vi "SeqeunceDefinitionDialog.vi"(11 "TestSequence":T3[](array[typedef])) -> (1 "TestSequence out":T3[](array[typedef]), 3 "Cancelled?":bool=TRUE)   [LabVIEW 2017]
doc: "Use this template to create a dialog box with event handling."
uses:
  ModuleUICluster.ctl
  TestStep-StepType.ctl
  TestStepTypes.ctl
  RF Direction.ctl
  PolarizationSelect.ctl
panel:
  in  "Save As File":bool
  in  "Load File":bool
  in  "tab":T1(tab)
  in  "module 7":T2={"Tx Vertical"=FALSE, "Tx Horizontal"=FALSE, "Rx Vertical"=FALSE, "Rx Horizontal"=FALSE, "Attenuation, dB"=[63], "Phase Shift, deg"=[64]}
  in  "module 6":T2={"Tx Vertical"=FALSE, "Tx Horizontal"=FALSE, "Rx Vertical"=FALSE, "Rx Horizontal"=FALSE, "Attenuation, dB"=[63], "Phase Shift, deg"=[64]}
  in  "module 5":T2={"Tx Vertical"=FALSE, "Tx Horizontal"=FALSE, "Rx Vertical"=FALSE, "Rx Horizontal"=FALSE, "Attenuation, dB"=[63], "Phase Shift, deg"=[64]}
  in  "module 4":T2={"Tx Vertical"=FALSE, "Tx Horizontal"=FALSE, "Rx Vertical"=FALSE, "Rx Horizontal"=FALSE, "Attenuation, dB"=[63], "Phase Shift, deg"=[64]}
  in  "module 3":T2={"Tx Vertical"=FALSE, "Tx Horizontal"=FALSE, "Rx Vertical"=FALSE, "Rx Horizontal"=FALSE, "Attenuation, dB"=[63], "Phase Shift, deg"=[64]}
  in  "module 2":T2={"Tx Vertical"=FALSE, "Tx Horizontal"=FALSE, "Rx Vertical"=FALSE, "Rx Horizontal"=FALSE, "Attenuation, dB"=[63], "Phase Shift, deg"=[64]}
  in  "module 1":T2={"Tx Vertical"=FALSE, "Tx Horizontal"=FALSE, "Rx Vertical"=FALSE, "Rx Horizontal"=FALSE, "Attenuation, dB"=[63], "Phase Shift, deg"=[64]}
  in  "module 0":T2={"Tx Vertical"=FALSE, "Tx Horizontal"=FALSE, "Rx Vertical"=FALSE, "Rx Horizontal"=FALSE, "Attenuation, dB"=[63], "Phase Shift, deg"=[64]}
  in  "module 8":T2={"Tx Vertical"=FALSE, "Tx Horizontal"=FALSE, "Rx Vertical"=FALSE, "Rx Horizontal"=FALSE, "Attenuation, dB"=[63], "Phase Shift, deg"=[64]}
  in  "module 9":T2={"Tx Vertical"=FALSE, "Tx Horizontal"=FALSE, "Rx Vertical"=FALSE, "Rx Horizontal"=FALSE, "Attenuation, dB"=[63], "Phase Shift, deg"=[64]}
  in  "module 10":T2={"Tx Vertical"=FALSE, "Tx Horizontal"=FALSE, "Rx Vertical"=FALSE, "Rx Horizontal"=FALSE, "Attenuation, dB"=[63], "Phase Shift, deg"=[64]}
  in  "module 11":T2={"Tx Vertical"=FALSE, "Tx Horizontal"=FALSE, "Rx Vertical"=FALSE, "Rx Horizontal"=FALSE, "Attenuation, dB"=[63], "Phase Shift, deg"=[64]}
  in  "module 12":T2={"Tx Vertical"=FALSE, "Tx Horizontal"=FALSE, "Rx Vertical"=FALSE, "Rx Horizontal"=FALSE, "Attenuation, dB"=[63], "Phase Shift, deg"=[64]}
  in  "module 13":T2={"Tx Vertical"=FALSE, "Tx Horizontal"=FALSE, "Rx Vertical"=FALSE, "Rx Horizontal"=FALSE, "Attenuation, dB"=[63], "Phase Shift, deg"=[64]}
  in  "module 14":T2={"Tx Vertical"=FALSE, "Tx Horizontal"=FALSE, "Rx Vertical"=FALSE, "Rx Horizontal"=FALSE, "Attenuation, dB"=[63], "Phase Shift, deg"=[64]}
  in  "module 15":T2={"Tx Vertical"=FALSE, "Tx Horizontal"=FALSE, "Rx Vertical"=FALSE, "Rx Horizontal"=FALSE, "Attenuation, dB"=[63], "Phase Shift, deg"=[64]}
  in  "module 23":T2={"Tx Vertical"=FALSE, "Tx Horizontal"=FALSE, "Rx Vertical"=FALSE, "Rx Horizontal"=FALSE, "Attenuation, dB"=[63], "Phase Shift, deg"=[64]}
  in  "module 22":T2={"Tx Vertical"=FALSE, "Tx Horizontal"=FALSE, "Rx Vertical"=FALSE, "Rx Horizontal"=FALSE, "Attenuation, dB"=[63], "Phase Shift, deg"=[64]}
  in  "module 21":T2={"Tx Vertical"=FALSE, "Tx Horizontal"=FALSE, "Rx Vertical"=FALSE, "Rx Horizontal"=FALSE, "Attenuation, dB"=[63], "Phase Shift, deg"=[64]}
  in  "module 20":T2={"Tx Vertical"=FALSE, "Tx Horizontal"=FALSE, "Rx Vertical"=FALSE, "Rx Horizontal"=FALSE, "Attenuation, dB"=[63], "Phase Shift, deg"=[64]}
  in  "module 19":T2={"Tx Vertical"=FALSE, "Tx Horizontal"=FALSE, "Rx Vertical"=FALSE, "Rx Horizontal"=FALSE, "Attenuation, dB"=[63], "Phase Shift, deg"=[64]}
  in  "module 18":T2={"Tx Vertical"=FALSE, "Tx Horizontal"=FALSE, "Rx Vertical"=FALSE, "Rx Horizontal"=FALSE, "Attenuation, dB"=[63], "Phase Shift, deg"=[64]}
  in  "module 17":T2={"Tx Vertical"=FALSE, "Tx Horizontal"=FALSE, "Rx Vertical"=FALSE, "Rx Horizontal"=FALSE, "Attenuation, dB"=[63], "Phase Shift, deg"=[64]}
  in  "module 16":T2={"Tx Vertical"=FALSE, "Tx Horizontal"=FALSE, "Rx Vertical"=FALSE, "Rx Horizontal"=FALSE, "Attenuation, dB"=[63], "Phase Shift, deg"=[64]}
  in  "module 31":T2={"Tx Vertical"=FALSE, "Tx Horizontal"=FALSE, "Rx Vertical"=FALSE, "Rx Horizontal"=FALSE, "Attenuation, dB"=[63], "Phase Shift, deg"=[64]}
  in  "module 30":T2={"Tx Vertical"=FALSE, "Tx Horizontal"=FALSE, "Rx Vertical"=FALSE, "Rx Horizontal"=FALSE, "Attenuation, dB"=[63], "Phase Shift, deg"=[64]}
  in  "module 29":T2={"Tx Vertical"=FALSE, "Tx Horizontal"=FALSE, "Rx Vertical"=FALSE, "Rx Horizontal"=FALSE, "Attenuation, dB"=[63], "Phase Shift, deg"=[64]}
  in  "module 28":T2={"Tx Vertical"=FALSE, "Tx Horizontal"=FALSE, "Rx Vertical"=FALSE, "Rx Horizontal"=FALSE, "Attenuation, dB"=[63], "Phase Shift, deg"=[64]}
  in  "module 27":T2={"Tx Vertical"=FALSE, "Tx Horizontal"=FALSE, "Rx Vertical"=FALSE, "Rx Horizontal"=FALSE, "Attenuation, dB"=[63], "Phase Shift, deg"=[64]}
  in  "module 26":T2={"Tx Vertical"=FALSE, "Tx Horizontal"=FALSE, "Rx Vertical"=FALSE, "Rx Horizontal"=FALSE, "Attenuation, dB"=[63], "Phase Shift, deg"=[64]}
  in  "module 25":T2={"Tx Vertical"=FALSE, "Tx Horizontal"=FALSE, "Rx Vertical"=FALSE, "Rx Horizontal"=FALSE, "Attenuation, dB"=[63], "Phase Shift, deg"=[64]}
  in  "module 24":T2={"Tx Vertical"=FALSE, "Tx Horizontal"=FALSE, "Rx Vertical"=FALSE, "Rx Horizontal"=FALSE, "Attenuation, dB"=[63], "Phase Shift, deg"=[64]}
  in  "module 39":T2={"Tx Vertical"=FALSE, "Tx Horizontal"=FALSE, "Rx Vertical"=FALSE, "Rx Horizontal"=FALSE, "Attenuation, dB"=[63], "Phase Shift, deg"=[64]}
  in  "module 38":T2={"Tx Vertical"=FALSE, "Tx Horizontal"=FALSE, "Rx Vertical"=FALSE, "Rx Horizontal"=FALSE, "Attenuation, dB"=[63], "Phase Shift, deg"=[64]}
  in  "module 37":T2={"Tx Vertical"=FALSE, "Tx Horizontal"=FALSE, "Rx Vertical"=FALSE, "Rx Horizontal"=FALSE, "Attenuation, dB"=[63], "Phase Shift, deg"=[64]}
  in  "module 36":T2={"Tx Vertical"=FALSE, "Tx Horizontal"=FALSE, "Rx Vertical"=FALSE, "Rx Horizontal"=FALSE, "Attenuation, dB"=[63], "Phase Shift, deg"=[64]}
  in  "module 35":T2={"Tx Vertical"=FALSE, "Tx Horizontal"=FALSE, "Rx Vertical"=FALSE, "Rx Horizontal"=FALSE, "Attenuation, dB"=[63], "Phase Shift, deg"=[64]}
  in  "module 34":T2={"Tx Vertical"=FALSE, "Tx Horizontal"=FALSE, "Rx Vertical"=FALSE, "Rx Horizontal"=FALSE, "Attenuation, dB"=[63], "Phase Shift, deg"=[64]}
  in  "module 33":T2={"Tx Vertical"=FALSE, "Tx Horizontal"=FALSE, "Rx Vertical"=FALSE, "Rx Horizontal"=FALSE, "Attenuation, dB"=[63], "Phase Shift, deg"=[64]}
  in  "module 32":T2={"Tx Vertical"=FALSE, "Tx Horizontal"=FALSE, "Rx Vertical"=FALSE, "Rx Horizontal"=FALSE, "Attenuation, dB"=[63], "Phase Shift, deg"=[64]}
  in  "module 47":T2={"Tx Vertical"=FALSE, "Tx Horizontal"=FALSE, "Rx Vertical"=FALSE, "Rx Horizontal"=FALSE, "Attenuation, dB"=[63], "Phase Shift, deg"=[64]}
  in  "module 46":T2={"Tx Vertical"=FALSE, "Tx Horizontal"=FALSE, "Rx Vertical"=FALSE, "Rx Horizontal"=FALSE, "Attenuation, dB"=[63], "Phase Shift, deg"=[64]}
  in  "module 45":T2={"Tx Vertical"=FALSE, "Tx Horizontal"=FALSE, "Rx Vertical"=FALSE, "Rx Horizontal"=FALSE, "Attenuation, dB"=[63], "Phase Shift, deg"=[64]}
  in  "module 44":T2={"Tx Vertical"=FALSE, "Tx Horizontal"=FALSE, "Rx Vertical"=FALSE, "Rx Horizontal"=FALSE, "Attenuation, dB"=[63], "Phase Shift, deg"=[64]}
  in  "module 43":T2={"Tx Vertical"=FALSE, "Tx Horizontal"=FALSE, "Rx Vertical"=FALSE, "Rx Horizontal"=FALSE, "Attenuation, dB"=[63], "Phase Shift, deg"=[64]}
  in  "module 42":T2={"Tx Vertical"=FALSE, "Tx Horizontal"=FALSE, "Rx Vertical"=FALSE, "Rx Horizontal"=FALSE, "Attenuation, dB"=[63], "Phase Shift, deg"=[64]}
  in  "module 41":T2={"Tx Vertical"=FALSE, "Tx Horizontal"=FALSE, "Rx Vertical"=FALSE, "Rx Horizontal"=FALSE, "Attenuation, dB"=[63], "Phase Shift, deg"=[64]}
  in  "module 40":T2={"Tx Vertical"=FALSE, "Tx Horizontal"=FALSE, "Rx Vertical"=FALSE, "Rx Horizontal"=FALSE, "Attenuation, dB"=[63], "Phase Shift, deg"=[64]}
  in  "module 55":T2={"Tx Vertical"=FALSE, "Tx Horizontal"=FALSE, "Rx Vertical"=FALSE, "Rx Horizontal"=FALSE, "Attenuation, dB"=[63], "Phase Shift, deg"=[64]}
  in  "module 54":T2={"Tx Vertical"=FALSE, "Tx Horizontal"=FALSE, "Rx Vertical"=FALSE, "Rx Horizontal"=FALSE, "Attenuation, dB"=[63], "Phase Shift, deg"=[64]}
  in  "module 53":T2={"Tx Vertical"=FALSE, "Tx Horizontal"=FALSE, "Rx Vertical"=FALSE, "Rx Horizontal"=FALSE, "Attenuation, dB"=[63], "Phase Shift, deg"=[64]}
  in  "module 52":T2={"Tx Vertical"=FALSE, "Tx Horizontal"=FALSE, "Rx Vertical"=FALSE, "Rx Horizontal"=FALSE, "Attenuation, dB"=[63], "Phase Shift, deg"=[64]}
  in  "module 51":T2={"Tx Vertical"=FALSE, "Tx Horizontal"=FALSE, "Rx Vertical"=FALSE, "Rx Horizontal"=FALSE, "Attenuation, dB"=[63], "Phase Shift, deg"=[64]}
  in  "module 50":T2={"Tx Vertical"=FALSE, "Tx Horizontal"=FALSE, "Rx Vertical"=FALSE, "Rx Horizontal"=FALSE, "Attenuation, dB"=[63], "Phase Shift, deg"=[64]}
  in  "module 49":T2={"Tx Vertical"=FALSE, "Tx Horizontal"=FALSE, "Rx Vertical"=FALSE, "Rx Horizontal"=FALSE, "Attenuation, dB"=[63], "Phase Shift, deg"=[64]}
  in  "module 48":T2={"Tx Vertical"=FALSE, "Tx Horizontal"=FALSE, "Rx Vertical"=FALSE, "Rx Horizontal"=FALSE, "Attenuation, dB"=[63], "Phase Shift, deg"=[64]}
  in  "module 63":T2={"Tx Vertical"=FALSE, "Tx Horizontal"=FALSE, "Rx Vertical"=FALSE, "Rx Horizontal"=FALSE, "Attenuation, dB"=[63], "Phase Shift, deg"=[64]}
  in  "module 62":T2={"Tx Vertical"=FALSE, "Tx Horizontal"=FALSE, "Rx Vertical"=FALSE, "Rx Horizontal"=FALSE, "Attenuation, dB"=[63], "Phase Shift, deg"=[64]}
  in  "module 61":T2={"Tx Vertical"=FALSE, "Tx Horizontal"=FALSE, "Rx Vertical"=FALSE, "Rx Horizontal"=FALSE, "Attenuation, dB"=[63], "Phase Shift, deg"=[64]}
  in  "module 60":T2={"Tx Vertical"=FALSE, "Tx Horizontal"=FALSE, "Rx Vertical"=FALSE, "Rx Horizontal"=FALSE, "Attenuation, dB"=[63], "Phase Shift, deg"=[64]}
  in  "module 59":T2={"Tx Vertical"=FALSE, "Tx Horizontal"=FALSE, "Rx Vertical"=FALSE, "Rx Horizontal"=FALSE, "Attenuation, dB"=[63], "Phase Shift, deg"=[64]}
  in  "module 58":T2={"Tx Vertical"=FALSE, "Tx Horizontal"=FALSE, "Rx Vertical"=FALSE, "Rx Horizontal"=FALSE, "Attenuation, dB"=[63], "Phase Shift, deg"=[64]}
  in  "module 57":T2={"Tx Vertical"=FALSE, "Tx Horizontal"=FALSE, "Rx Vertical"=FALSE, "Rx Horizontal"=FALSE, "Attenuation, dB"=[63], "Phase Shift, deg"=[64]}
  in  "module 56":T2={"Tx Vertical"=FALSE, "Tx Horizontal"=FALSE, "Rx Vertical"=FALSE, "Rx Horizontal"=FALSE, "Attenuation, dB"=[63], "Phase Shift, deg"=[64]}
  in  "De-Select All":bool
  in  "Select All":bool
  in  "Cancel":bool
  in  "OK":bool
  # "Module 0"
  # "Module 1"
  # "Module 2"
  # "Module 3"
  # "Module 4"
  # "Module 5"
  # "Module 6"
  # "Module 7"
  # "Module 8"
  # "Module 9"
  # "Module 10"
  # "Module 11"
  # "Module 12"
  # "Module 13"
  # "Module 14"
  # "Module 15"
  # "Module 16"
  # "Module 17"
  # "Module 18"
  # "Module 19"
  # "Module 20"
  # "Module 21"
  # "Module 22"
  # "Module 23"
  # "Module 24"
  # "Module 25"
  # "Module 26"
  # "Module 27"
  # "Module 28"
  # "Module 29"
  # "Module 30"
  # "Module 31"
  # "Module 32"
  # "Module 33"
  # "Module 34"
  # "Module 35"
  # "Module 36"
  # "Module 37"
  # "Module 38"
  # "Module 39"
  # "Module 40"
  # "Module 41"
  # "Module 42"
  # "Module 43"
  # "Module 44"
  # "Module 45"
  # "Module 46"
  # "Module 47"
  # "Module 48"
  # "Module 49"
  # "Module 50"
  # "Module 51"
  # "Module 52"
  # "Module 53"
  # "Module 54"
  # "Module 55"
  # "Module 56"
  # "Module 57"
  # "Module 58"
  # "Module 59"
  # "Module 60"
  # "Module 61"
  # "Module 62"
  # "Module 63"
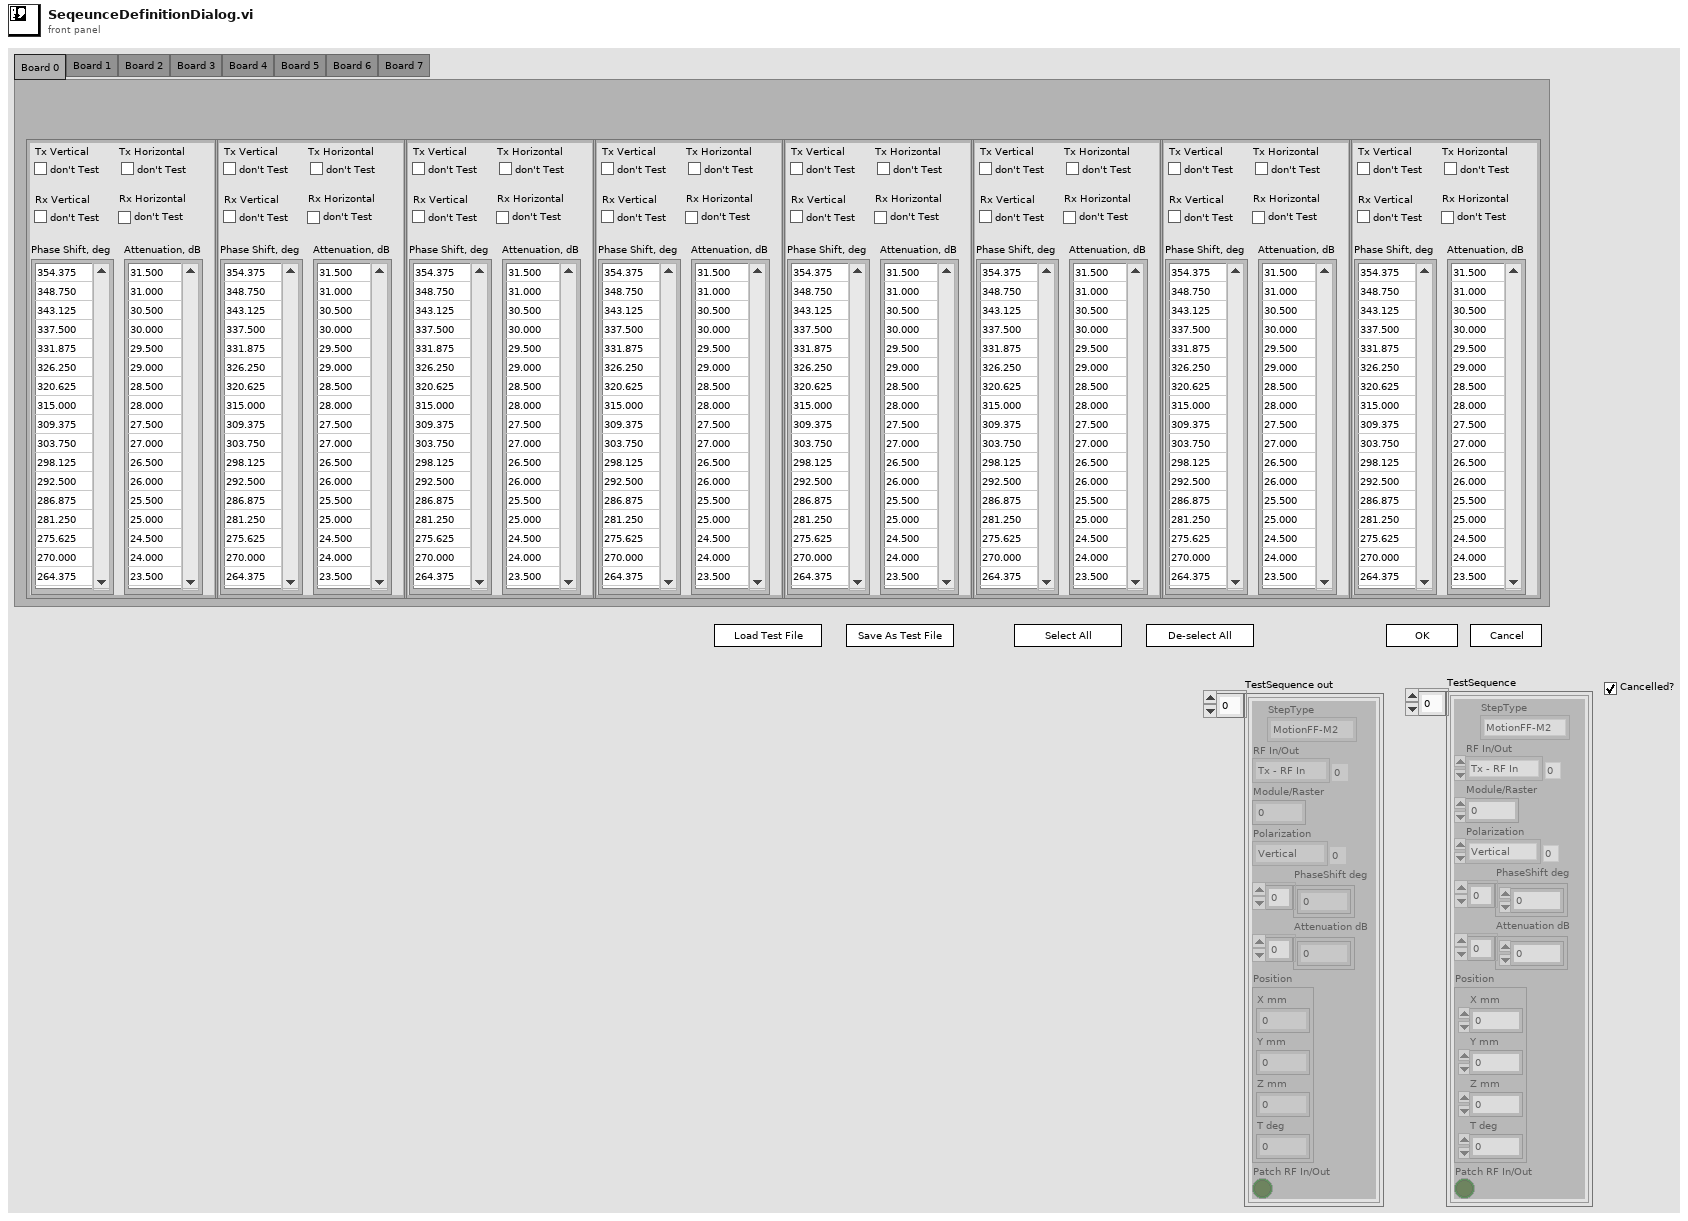
[diagram p1: front panel]
types:
  T1 = enum32{"Board 0", "Board 1", "Board 2", "Board 3", "Board 4", "Board 5", "Board 6", "Board 7"}
  T2 = typedef "ModuleUICluster.ctl" = cluster{"Tx Vertical":bool, "Tx Horizontal":bool, "Rx Vertical":bool, "Rx Horizontal":bool, "Attenuation, dB":i32[], "Phase Shift, deg":i32[]}
  T3 = typedef "TestStep-StepType.ctl" = cluster{"StepType":T4, "RF In/Out":T5, "Module/Raster":i32, "Polarization":T6, "PhaseShift deg":dbl[], "Attenuation dB":dbl[], "Position":cluster{"X mm":dbl, "Y mm":dbl, "Z mm":dbl, "T deg":dbl}, "Patch RF In/Out":bool}
  T4 = typedef "TestStepTypes.ctl" = enum16{"MotionFF-M2", "Motion", "SweepTest", "RasterTest", "Finish", "64ModuleCfg"}
  T5 = typedef "RF Direction.ctl" = enum16{"Tx - RF In", "Rx - RF Out"}
  T6 = typedef "PolarizationSelect.ctl" = enum16{"Vertical", "Horizontal"}
  T7 = cluster{"Tx Vertical":bool, "Tx Horizontal":bool, "Rx Vertical":bool, "Rx Horizontal":bool, "Attenuation, dB":i32[], "Phase Shift, deg":i32[]}
  T8 = enum16{"open", "replace", "create", "open or create", "replace or create", "replace or create with confirmation"}
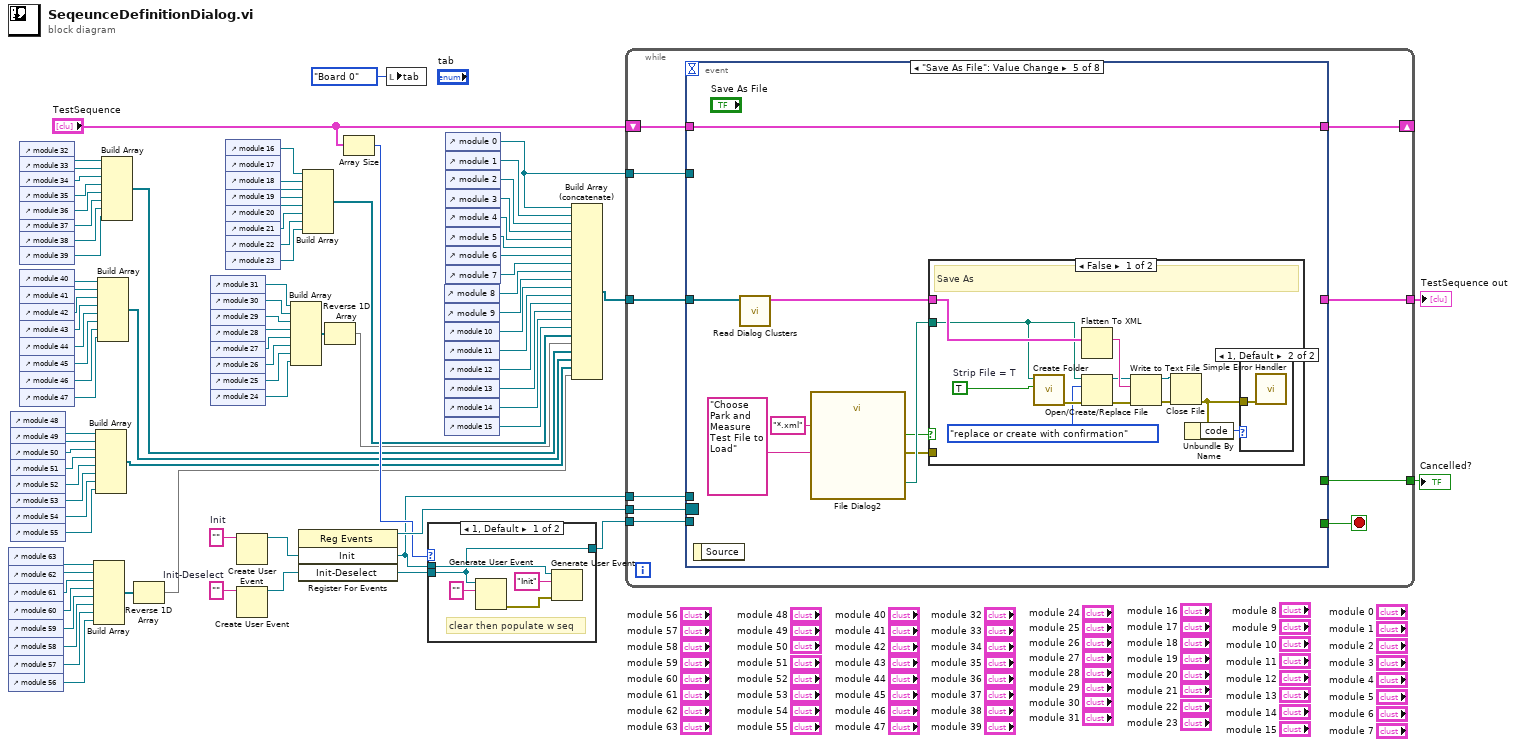
[diagram p0: block diagram]
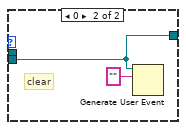
[diagram p2: hidden frame]
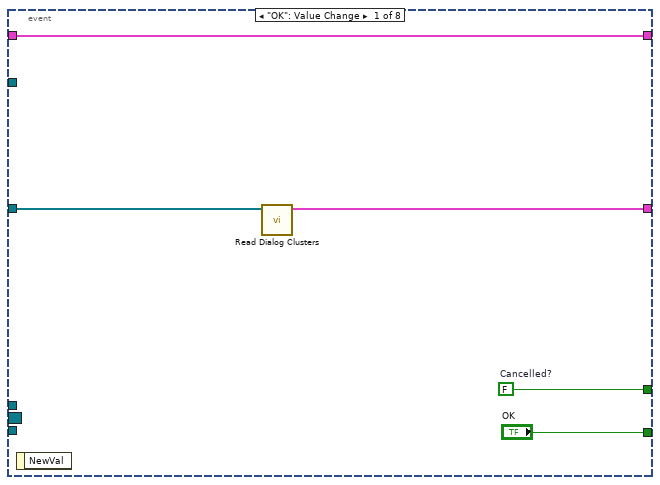
[diagram p3: hidden frame]
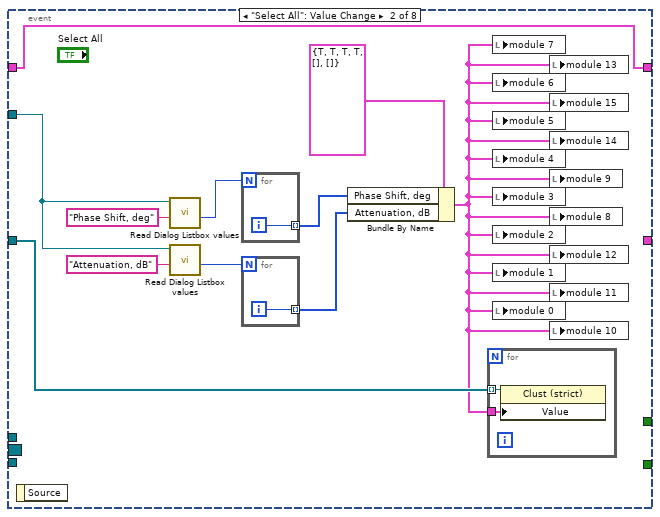
[diagram p4: hidden frame]
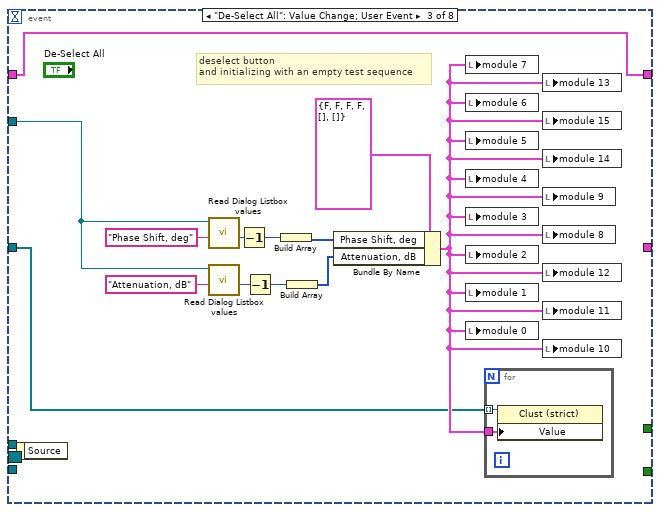
[diagram p5: hidden frame]
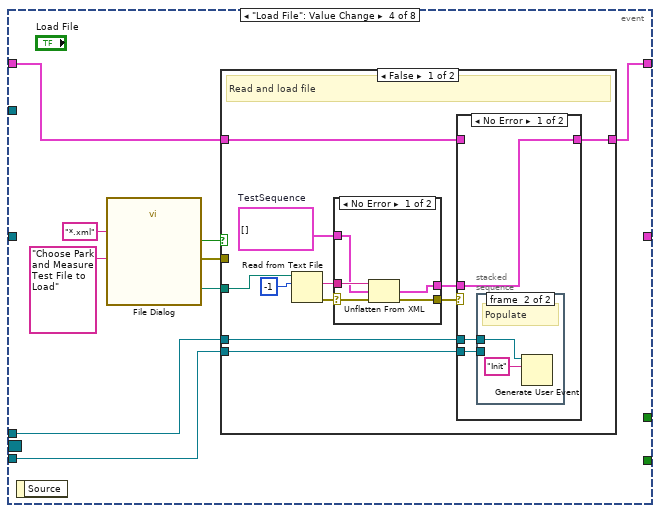
[diagram p6: hidden frame]
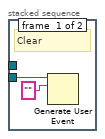
[diagram p7: hidden frame]
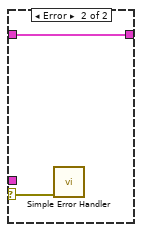
[diagram p8: hidden frame]
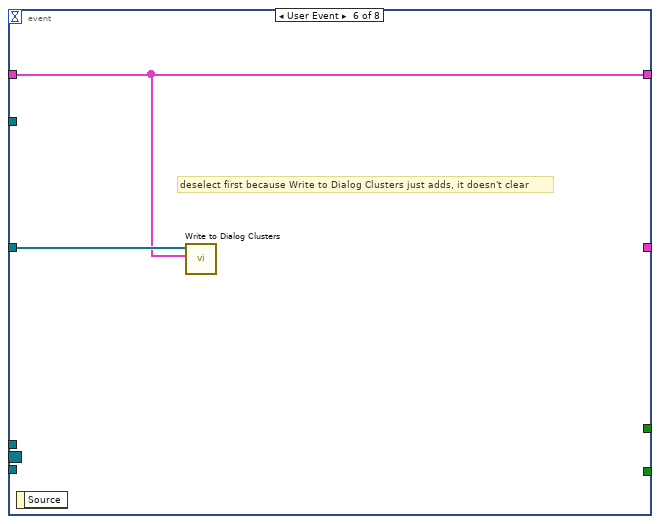
[diagram p13: hidden frame]
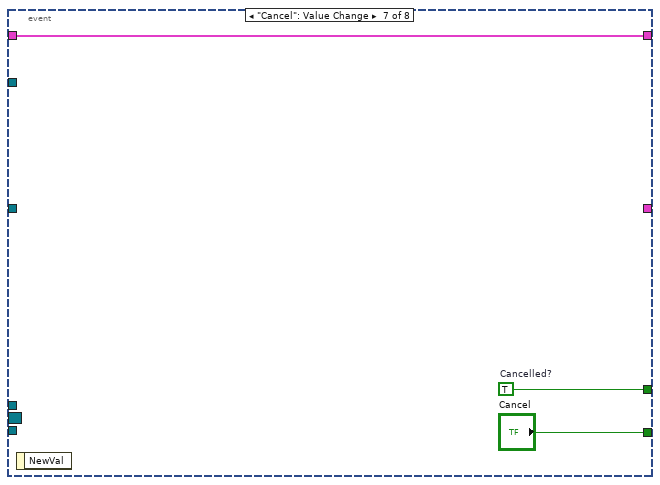
[diagram p14: hidden frame]
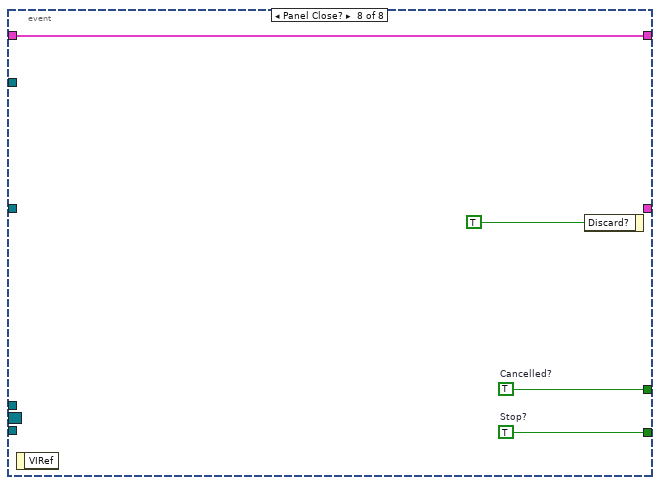
[diagram p15: hidden frame]
diagram:
  w71 = ""  # Init-Deselect
  w82 = ""  # Init
  n1 = control-ref of="module 63"() -> (w13:refnum<vi>)
  n2 = control-ref of="module 62"() -> (w12:refnum<vi>)
  n3 = control-ref of="module 61"() -> (w11:refnum<vi>)
  n4 = control-ref of="module 60"() -> (w10:refnum<vi>)
  n5 = control-ref of="module 59"() -> (w9:refnum<vi>)
  n6 = control-ref of="module 58"() -> (w8:refnum<vi>)
  n7 = control-ref of="module 57"() -> (w7:refnum<vi>)
  n8 = control-ref of="module 56"() -> (w6:refnum<vi>)
  n9 = control-ref of="module 48"() -> (w22:refnum<vi>)
  n10 = control-ref of="module 49"() -> (w21:refnum<vi>)
  n11 = control-ref of="module 50"() -> (w20:refnum<vi>)
  n12 = control-ref of="module 51"() -> (w19:refnum<vi>)
  n13 = control-ref of="module 52"() -> (w18:refnum<vi>)
  n14 = control-ref of="module 53"() -> (w17:refnum<vi>)
  n15 = control-ref of="module 54"() -> (w16:refnum<vi>)
  n16 = control-ref of="module 55"() -> (w15:refnum<vi>)
  n17 = control-ref of="module 32"() -> (w40:refnum<vi>)
  n18 = control-ref of="module 33"() -> (w39:refnum<vi>)
  n19 = control-ref of="module 34"() -> (w38:refnum<vi>)
  n20 = control-ref of="module 35"() -> (w37:refnum<vi>)
  n21 = control-ref of="module 36"() -> (w36:refnum<vi>)
  n22 = control-ref of="module 37"() -> (w33:refnum<vi>)
  n23 = control-ref of="module 38"() -> (w35:refnum<vi>)
  n24 = control-ref of="module 39"() -> (w34:refnum<vi>)
  n25 = control-ref of="module 40"() -> (w31:refnum<vi>)
  n26 = control-ref of="module 41"() -> (w30:refnum<vi>)
  n27 = control-ref of="module 42"() -> (w29:refnum<vi>)
  n28 = control-ref of="module 43"() -> (w28:refnum<vi>)
  n29 = control-ref of="module 44"() -> (w27:refnum<vi>)
  n30 = control-ref of="module 45"() -> (w26:refnum<vi>)
  n31 = control-ref of="module 46"() -> (w25:refnum<vi>)
  n32 = control-ref of="module 47"() -> (w24:refnum<vi>)
  n33 = Build Array(w13, w12, w11, w10, w9, w8, w7, w6) -> (w5:refnum<vi>[])
  n34 = Build Array(w22, w21, w20, w19, w18, w17, w16, w15) -> (w14:refnum<vi>[])
  n35 = Build Array(w31, w30, w29, w28, w27, w26, w25, w24) -> (w23:refnum<vi>[])
  n36 = Build Array(w40, w39, w38, w37, w36, w33, w35, w34) -> (w32:refnum<vi>[])
  n37 = Reverse 1D Array(array=w5) -> (reversed array=w4:refnum<vi>[])
  n38 = control-ref of="module 31"() -> (w50:refnum<vi>)
  n39 = control-ref of="module 30"() -> (w49:refnum<vi>)
  n40 = control-ref of="module 29"() -> (w48:refnum<vi>)
  n41 = control-ref of="module 28"() -> (w47:refnum<vi>)
  n42 = control-ref of="module 27"() -> (w46:refnum<vi>)
  n43 = control-ref of="module 26"() -> (w45:refnum<vi>)
  n44 = control-ref of="module 25"() -> (w44:refnum<vi>)
  n45 = control-ref of="module 24"() -> (w43:refnum<vi>)
  n46 = control-ref of="module 16"() -> (w60:refnum<vi>)
  n47 = control-ref of="module 17"() -> (w59:refnum<vi>)
  n48 = control-ref of="module 18"() -> (w58:refnum<vi>)
  n49 = control-ref of="module 19"() -> (w57:refnum<vi>)
  n50 = control-ref of="module 20"() -> (w56:refnum<vi>)
  n51 = control-ref of="module 21"() -> (w55:refnum<vi>)
  n52 = control-ref of="module 22"() -> (w54:refnum<vi>)
  n53 = control-ref of="module 23"() -> (w53:refnum<vi>)
  n54 = Create User Event(user event datatype=w82) -> (user event=w2:refnum<user-event>)  [unwired: 1 in, 1 out]
  n55 = Create User Event(user event datatype=w71) -> (user event=w70:refnum<user-event>)  [unwired: 1 in, 1 out]
  n56 = Build Array(w50, w49, w48, w47, w46, w45, w44, w43) -> (w42:refnum<vi>[])
  n57 = register-events(w2, w70) -> (reference out=w81:refnum<event-registration>)  [unwired: 2 in, 1 out]
  n58 = Build Array(w60, w59, w58, w57, w56, w55, w54, w53) -> (w51:refnum<vi>[])
  n59 = Reverse 1D Array(array=w42) -> (reversed array=w41:refnum<vi>[])
  n60 = Array Size(array="TestSequence") -> (size(s)=w52:i32)
  n61 = local write "tab"(enum32{"Board 0", "Board 1"}."Board 0" ("tab")) -> ()
  n62 = case shown="1, Default" w52 {
    tunnel: w2 -> [w89 _]
    tunnel: w70 -> [w85 w90]
    tunnel: [w85 w90] -> w3
    frame 1, Default {
      # "clear then populate w seq"
      n63 = Generate User Event(user event=w85, event data cluster="" ("event data")) -> (error out=w86:errorcluster)  [unwired: 2 in, 1 out]
      n64 = Generate User Event(user event=w89, event data cluster="Init" ("event data"), error in=w86) -> ()  [unwired: 1 in, 2 out]
    }
    frame 0 {
      # "clear"
      n65 = Generate User Event(user event=w90, event data cluster="" ("event data")) -> ()  [unwired: 2 in, 2 out]
    }
  }
  n66 = control-ref of="module 8"() -> (w68:refnum<vi>)
  n67 = control-ref of="module 9"() -> (w67:refnum<vi>)
  n68 = control-ref of="module 10"() -> (w66:refnum<vi>)
  n69 = control-ref of="module 11"() -> (w65:refnum<vi>)
  n70 = control-ref of="module 12"() -> (w64:refnum<vi>)
  n71 = control-ref of="module 13"() -> (w63:refnum<vi>)
  n72 = control-ref of="module 14"() -> (w62:refnum<vi>)
  n73 = control-ref of="module 15"() -> (w61:refnum<vi>)
  n74 = control-ref of="module 0"() -> (w73:refnum<vi>)
  n75 = control-ref of="module 1"() -> (w80:refnum<vi>)
  n76 = control-ref of="module 2"() -> (w79:refnum<vi>)
  n77 = control-ref of="module 3"() -> (w78:refnum<vi>)
  n78 = control-ref of="module 4"() -> (w77:refnum<vi>)
  n79 = control-ref of="module 5"() -> (w76:refnum<vi>)
  n80 = control-ref of="module 6"() -> (w75:refnum<vi>)
  n81 = control-ref of="module 7"() -> (w74:refnum<vi>)
  n82 = Build Array (concatenate)(w73, w80, w79, w78, w77, w76, w75, w74, w68, w67, w66, w65, w64, w63, w62, w61, w51, w41, w32, w23, w14, w4) -> (w72:refnum<vi>[])
  n83 = while {
    tunnel: [w100] -> w84
    tunnel: [w99] -> w83
    tunnel: w73 -> [w98]
    tunnel: w81 -> [w97]
    tunnel: w72 -> [w96]
    tunnel: w3 -> [w95]
    tunnel: w2 -> [w94]
    shift-right: [w92] -> _
    shift-left: "TestSequence" -> [w93]
    stop <- w101 stop-if-true
    n84 = event shown="[4] \"Save As File\": Value Change" {
      selector: w97 -> [_ _ _ _ _ _ _ _]
      dyn-events: _ -> [_ _ _ _ _ _ _ _]
      timeout: _ -> [_ _ _ _ _ _ _ _]
      tunnel: ["OK" _ _ _ _ _ "Cancel" w200] -> w101
      tunnel: [w106 _ _ _ _ _ w197 w199] -> w100
      tunnel: [w104 _ _ _ _ _ _ _] -> w99
      tunnel: w98 -> [_ w114 w132 _ _ _ _ _]
      tunnel: w96 -> [w103 w109 w123 _ w177 w194 _ _]
      tunnel: w93 -> [w102 w107 w122 w138 w172 w193 w195 w198]
      tunnel: w95 -> [_ _ _ w140 _ _ _ _]
      tunnel: w94 -> [_ _ _ w139 _ _ _ _]
      tunnel: [w102 w107 w122 w137 w172 w193 w195 w198] -> w92
      event "OK": Value Change {
        w106 = FALSE  # Cancelled?
        n85 = event-data() -> ()  [unwired: 1 in, 1 out]
        n86 = call "Read Dialog Clusters.vi"("Module Cluster Refs"=w103) -> ("TestSequence"=w104:T3[])  [unwired: 10 in]
      }
      event "Select All": Value Change {
        n87 = event-data() -> ()  [unwired: 1 in, 1 out]
        n88 = call "Read Dialog Listbox values.vi"("Label.Text"="Phase Shift, deg", "module ref"=w114) -> ("Names, len"=w113:i32)  [unwired: 8 in, 1 out]
        n89 = call "Read Dialog Listbox values.vi"("Label.Text"="Attenuation, dB", "module ref"=w114) -> ("Names, len"=w110:i32)  [unwired: 8 in, 1 out]
        n90 = for {
          N: w113 -> [_]
          tunnel: [w121] -> w116 mode=indexing
          i -> [w121]
        }
        n91 = for {
          N: w110 -> [_]
          tunnel: [w120] -> w112 mode=indexing
          i -> [w120]
        }
        n92 = Bundle By Name(cluster=T7 {"Tx Vertical"=TRUE, "Tx Horizontal"=TRUE, "Rx Vertical"=TRUE, "Rx Horizontal"=TRUE, "Attenuation, dB"=[], "Phase Shift, deg"=[]} ("module 0"), "Phase Shift, deg"=w116, "Attenuation, dB"=w112) -> (w108:T7)
        n93 = for {
          tunnel: w109 -> [w119] mode=indexing
          tunnel: w108 -> [w118]
          n94 = property class="Clust (strict)"(reference=w119, "Value"=w118) -> ()  [unwired: 1 in, 2 out]
        }
        n95 = local write "module 7"(w108) -> ()
        n96 = local write "module 6"(w108) -> ()
        n97 = local write "module 5"(w108) -> ()
        n98 = local write "module 4"(w108) -> ()
        n99 = local write "module 3"(w108) -> ()
        n100 = local write "module 2"(w108) -> ()
        n101 = local write "module 1"(w108) -> ()
        n102 = local write "module 0"(w108) -> ()
        n103 = local write "module 13"(w108) -> ()
        n104 = local write "module 15"(w108) -> ()
        n105 = local write "module 14"(w108) -> ()
        n106 = local write "module 9"(w108) -> ()
        n107 = local write "module 8"(w108) -> ()
        n108 = local write "module 12"(w108) -> ()
        n109 = local write "module 11"(w108) -> ()
        n110 = local write "module 10"(w108) -> ()
      }
      event "De-Select All": Value Change; User Event {
        # "deselect button\nand initializing with an empty test sequence"
        n111 = event-data() -> ()  [unwired: 1 in, 1 out]
        n112 = call "Read Dialog Listbox values.vi"("Label.Text"="Phase Shift, deg", "module ref"=w132) -> ("Names, len"=w130:i32)  [unwired: 8 in, 1 out]
        n113 = call "Read Dialog Listbox values.vi"("Label.Text"="Attenuation, dB", "module ref"=w132) -> ("Names, len"=w127:i32)  [unwired: 8 in, 1 out]
        n114 = Decrement(x=w130) -> (x-1=w129:i32)
        n115 = Decrement(x=w127) -> (x-1=w128:i32)
        n116 = Build Array(w129) -> (w125:i32[])
        n117 = Build Array(w128) -> (w126:i32[])
        n118 = Bundle By Name(cluster=T7 {"Tx Vertical"=FALSE, "Tx Horizontal"=FALSE, "Rx Vertical"=FALSE, "Rx Horizontal"=FALSE, "Attenuation, dB"=[], "Phase Shift, deg"=[]} ("module 0"), "Phase Shift, deg"=w125, "Attenuation, dB"=w126) -> (w124:T7)
        n119 = local write "module 7"(w124) -> ()
        n120 = local write "module 6"(w124) -> ()
        n121 = local write "module 5"(w124) -> ()
        n122 = local write "module 4"(w124) -> ()
        n123 = local write "module 3"(w124) -> ()
        n124 = local write "module 2"(w124) -> ()
        n125 = local write "module 1"(w124) -> ()
        n126 = local write "module 0"(w124) -> ()
        n127 = for {
          tunnel: w123 -> [w136] mode=indexing
          tunnel: w124 -> [w135]
          n128 = property class="Clust (strict)"(reference=w136, "Value"=w135) -> ()  [unwired: 1 in, 2 out]
        }
        n129 = local write "module 13"(w124) -> ()
        n130 = local write "module 15"(w124) -> ()
        n131 = local write "module 14"(w124) -> ()
        n132 = local write "module 9"(w124) -> ()
        n133 = local write "module 8"(w124) -> ()
        n134 = local write "module 12"(w124) -> ()
        n135 = local write "module 11"(w124) -> ()
        n136 = local write "module 10"(w124) -> ()
      }
      event "Load File": Value Change {
        n137 = event-data() -> ()  [unwired: 1 in, 1 out]
        n138 = call "File Dialog"("prompt"="Choose Park and Measure Test File to Load" ("default name"), "pattern (all files)"="*.xml") -> ("selected path"=w141:path, "cancelled"=w143:bool, "error out"=w142:errorcluster)  [unwired: 10 in, 1 out]
        n139 = case shown="False" w143 {
          tunnel: w142 -> [_ _]
          tunnel: w141 -> [w152 _]
          tunnel: w140 -> [w149 _]
          tunnel: w139 -> [w148 _]
          tunnel: [w147 w171] -> w137
          tunnel: w138 -> [w146 w171]
          frame False {
            w153 = T3[] []  # TestSequence
            # "Read and load file"
            n140 = Read from Text File(file (use dialog)=w152, count=-1) -> (text=w156:string, error out=w154:errorcluster)  [unwired: 2 in, 2 out]
            n141 = case shown="No Error" w154 {
              selector: w154 -> [w166 _]
              tunnel: w156 -> [w170 _]
              tunnel: w153 -> [w169 _]
              tunnel: [w168 _] -> w150
              tunnel: [w167 _] -> w151
              frame No Error {
                n142 = Unflatten From XML(xml string=w170, type=w169, error in (no error)=w166) -> (value=w168:T3[], error out=w167:errorcluster)
              }
              frame Error {
              }
            }
            n143 = case shown="No Error" w151 {
              selector: w151 -> [_ w165]
              tunnel: w150 -> [w157 _]
              tunnel: w149 -> [w159 _]
              tunnel: w148 -> [w158 _]
              tunnel: [w157 w164] -> w147
              tunnel: w146 -> [_ w164]
              frame No Error {
                n144 = stacked-sequence {
                  tunnel: w159 -> [w160 _]
                  tunnel: w158 -> [_ w162]
                  frame #0 {
                    # "Clear"
                    n145 = Generate User Event(user event=w160, event data cluster="" ("event data")) -> ()  [unwired: 2 in, 2 out]
                  }
                  frame #1 {
                    # "Populate"
                    n146 = Generate User Event(user event=w162, event data cluster="Init" ("event data")) -> ()  [unwired: 2 in, 2 out]
                  }
                }
              }
              frame Error {
                n147 = call <vilib>:"Simple Error Handler.vi"("error in (no error)"=w165) -> ()  [unwired: 4 in, 5 out]
              }
            }
          }
          frame True {
            # "Cancel"
          }
        }
      }
      event "Save As File": Value Change {
        n148 = event-data() -> ()  [unwired: 1 in, 1 out]
        n149 = call "Read Dialog Clusters.vi"("Module Cluster Refs"=w177) -> ("TestSequence"=w176:T3[])  [unwired: 10 in]
        n150 = call "File Dialog2"("prompt"="Choose Park and Measure Test File to Load" ("default name"), "pattern (all files)"="*.xml") -> ("selected path"=w175:path, "cancelled"=w174:bool, "error out"=w173:errorcluster)  [unwired: 10 in, 1 out]
        n151 = case shown="False" w174 {
          tunnel: w176 -> [w189 _]
          tunnel: w175 -> [w185 _]
          tunnel: w173 -> [_ _]
          frame False {
            w190 = TRUE  # Strip File = T
            # "Save As"
            n152 = call "Create Folder.vi"("Strip File = T"=w190, "Path"=w185) -> ("error out"=w187:errorcluster)  [unwired: 9 in]
            n153 = Flatten To XML(anything=w189) -> (xml string=w191:string)
            n154 = Open/Create/Replace File(file path (use dialog)=w185, error in=w187, operation (0:open)=T8."replace or create with confirmation") -> (refnum out=w184:refnum<file>, error out=w186:errorcluster)  [unwired: 3 in, 1 out]
            n155 = Write to Text File(file (use dialog)=w184, text=w191, error in=w186) -> (refnum out=w182:refnum<file>, error out=w188:errorcluster)  [unwired: 1 in, 1 out]
            n156 = Close File(refnum=w182, error in=w188) -> (error out=w181:errorcluster)  [unwired: 1 out]
            n157 = Unbundle By Name(w181) -> ("code"=w180:i32)
            n158 = case shown="1, Default" w180 {
              tunnel: w181 -> [_ w192]
              frame 43 {
              }
              frame 1, Default {
                n159 = call <vilib>:"Simple Error Handler.vi"("error in (no error)"=w192) -> ()  [unwired: 4 in, 5 out]
              }
            }
          }
          frame True {
            # "Cancel"
          }
        }
      }
      event User Event {
        # "deselect first because Write to Dialog Clusters just adds, it doesn't clear"
        n160 = event-data() -> ()  [unwired: 1 in, 1 out]
        n161 = call "Write to Dialog Clusters.vi"("TestSequence"=w193, "Module Cluster Refs"=w194) -> ()  [unwired: 10 in]
      }
      event "Cancel": Value Change {
        w197 = TRUE  # Cancelled?
        n162 = event-data() -> ()  [unwired: 1 in, 1 out]
      }
      event Panel Close? {
        w199 = TRUE  # Cancelled?
        w200 = TRUE  # Stop?
        n163 = event-data() -> ()  [unwired: 1 in, 1 out]
        n164 = event-data("Discard?"=TRUE) -> ()  [unwired: 1 in, 1 out]
      }
    }
  }
  "Cancelled?" <- w84
  "TestSequence out" <- w83
